vi "Enable-Disable Refs.vi"(9 "Enable/Disable":bool, 11 "Ctr Refs":refnum<vi>[](array[refnum])) -> ()   [LabVIEW 2015]
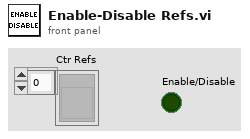
[diagram p1: front panel]
types:
  T1 = enum8{"Enabled", "Disabled", "Disabled and Grayed Out"}
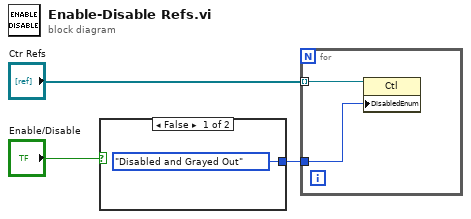
[diagram p0: block diagram]
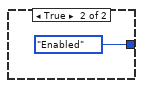
[diagram p2: hidden frame]
diagram:
  n1 = case shown="False" "Enable/Disable" {
    tunnel: [T1."Disabled and Grayed Out" ("Disabled") T1."Enabled" ("Disabled")] -> w1
    frame False {
    }
    frame True {
    }
  }
  n2 = for {
    tunnel: "Ctr Refs" -> [w7] mode=indexing
    tunnel: w1 -> [w6]
    n3 = property class="Ctl"(reference=w7, "DisabledEnum"=w6) -> ()  [unwired: 1 in, 2 out]
  }
